vi "camera.vi"() -> ()   [LabVIEW 2014]
uses:
  <vilib>/userdefined/High Color/IMAQdx.ctl
  <vilib>/vision/driver/NI_Vision_Acquisition_Software.lvlib
panel:
  out "Image 2":T1(plugin-control)
  out "Image":T1(plugin-control)
  in  "Session In":T2
  in  "stop":bool
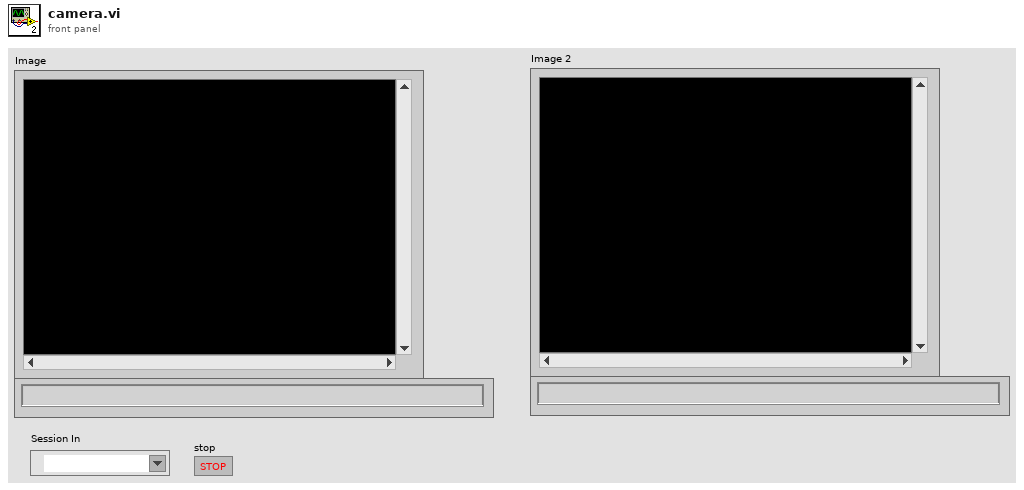
[diagram p1: front panel]
types:
  T1 = typedef "IMAQ Image.ctl" = refnum<image>
  T2 = typedef "IMAQdx.ctl" = refnum<k21>
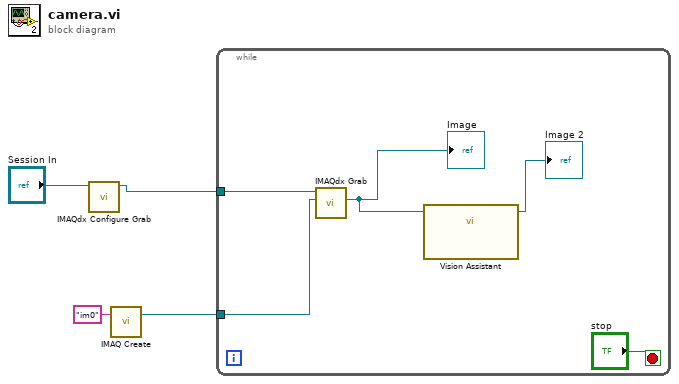
[diagram p0: block diagram]
diagram:
  n1 = call <vilib>:"IMAQdx Configure Grab.vi"("Session In"="Session In") -> ("Session Out"=w3:T2)  [unwired: 9 in, 1 out]
  n2 = call "IMAQ Create"("Image Name"="im0") -> ("New Image"=w2:T1)  [unwired: 4 in, 1 out]
  n3 = while {
    tunnel: w3 -> [w8]
    tunnel: w2 -> [w7]
    stop <- "stop" stop-if-true
    n4 = call <vilib>:"IMAQdx Grab.vi"("Image In"=w7, "Session In"=w8) -> ("Image Out"=w6:T1)  [unwired: 6 in, 3 out]
    "Image" <- w6
    n5 = call "Vision Assistant"("Image In"=w6) -> ("Image Out"=→"Image 2":T1)  [unwired: 25 in, 1 out]
  }
